vi "NanoStep InitAxis.vi"(6 "CtrlRef":T1 caption="Control Reference", 7 "AxeInv":bool, 8 "error in":errorcluster, 9 "Axis":u16(ring)=1 items=["Axis 0", "Axis 1"], 10 "Input Units":i8(ring) items=["mm", "ps"], 11 "VISA Rsrc":refnum<visa-resource-name>="NANOSTEP") -> (0 "error out":errorcluster, 2 "Pos Out":dbl=0.5)   [LabVIEW 2010]
uses:
  <userlib>/GenProg/WritebyRefBool.vi
  <userlib>/GenProg/ReadbyRefBool.vi
  <userlib>/GenProg/WritebyRefNum.vi
  <userlib>/NanoStep/NanoStep WaitMess.vi
panel:
  out "DatumDone":bool
  out "Canceled":bool
  in  "Annuler":bool
  out "ShowMess":bool
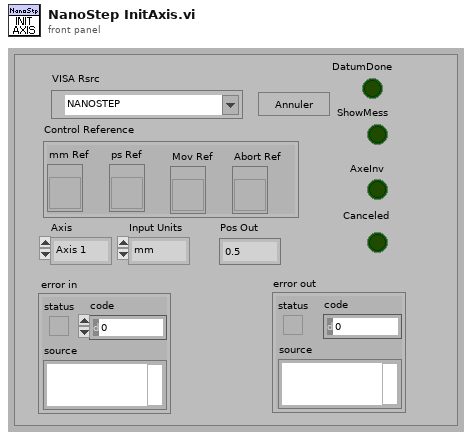
[diagram p1: front panel]
types:
  T1 = cluster{"mm Ref":refnum<vi>, "ps Ref":refnum<vi>, "Mov Ref":refnum<vi>, "Abort Ref":refnum<vi>}
  T2 = enum16{"Clear buffer", "Ack", "Datum", "read position", "end"}
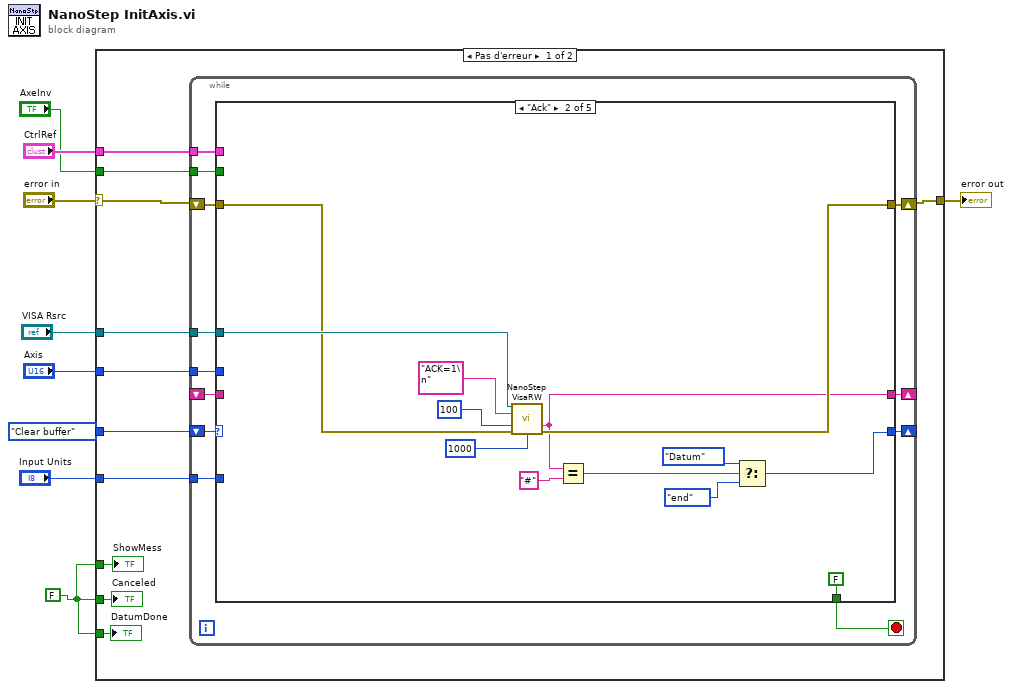
[diagram p0: block diagram]
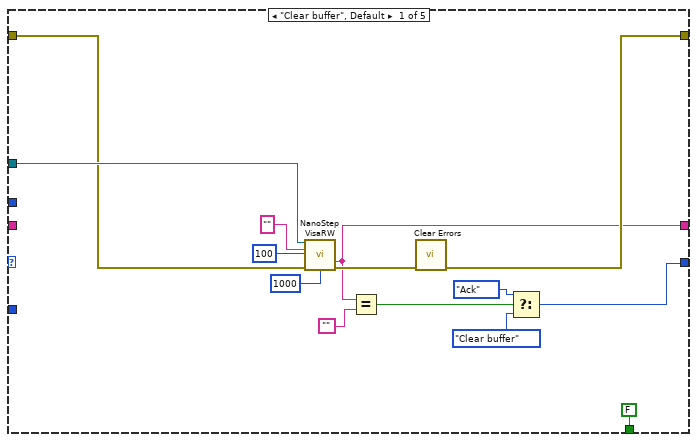
[diagram p2: hidden frame]
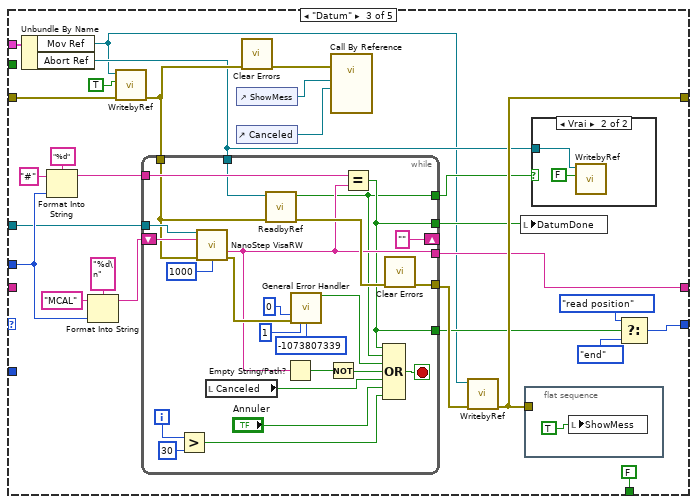
[diagram p3: hidden frame]
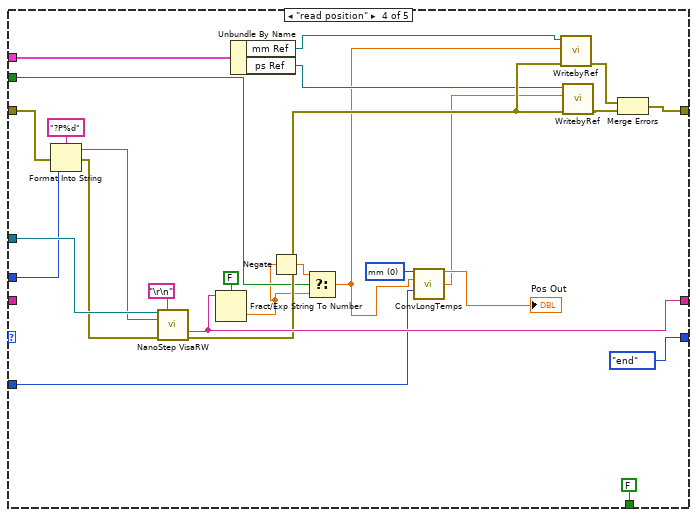
[diagram p5: hidden frame]
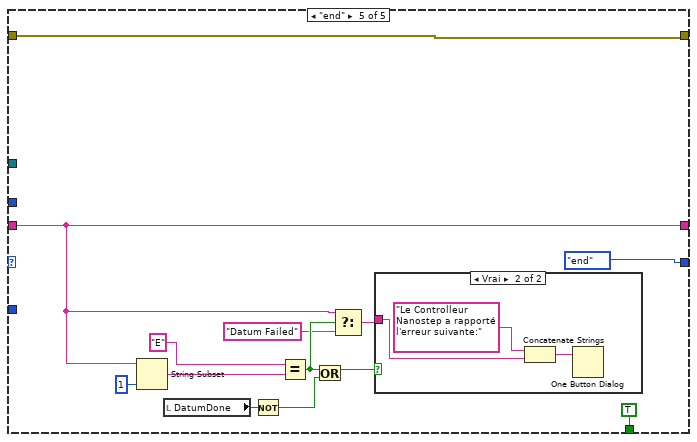
[diagram p6: hidden frame]
diagram:
  w4 = FALSE ("Canceled")
  n1 = case shown="Pas d'erreur" "error in" {
    selector: "error in" -> [w18 w157]
    tunnel: "Axis" -> [w20 _]
    tunnel: [w17 w157] -> w7
    tunnel: T2."Clear buffer" ("Énum") -> [w19 _]
    tunnel: "VISA Rsrc" -> [w16 _]
    tunnel: w4 -> [w15 _]
    tunnel: w4 -> [w14 _]
    tunnel: w4 -> [w13 _]
    tunnel: "CtrlRef" -> [w12 _]
    tunnel: "Input Units" -> [w11 _]
    tunnel: "AxeInv" -> [w10 _]
    frame No Error {
      n2 = while {
        tunnel: w20 -> [w32]
        shift-right: [w28] -> w17
        shift-left: w18 -> [w30]
        tunnel: w16 -> [w29]
        shift-right: [w26] -> _
        shift-left: w19 -> [w31]
        shift-right: [w25] -> _
        shift-left: _ -> [w24]
        tunnel: w12 -> [w23]
        tunnel: w11 -> [w22]
        tunnel: w10 -> [w21]
        stop <- w27 stop-if-true
        n3 = case shown="\"Ack\"" w31 {
          tunnel: w32 -> [_ _ w78 w138 _]
          tunnel: w30 -> [w43 w56 w77 w137 w152]
          tunnel: w29 -> [w46 w59 w72 w140 _]
          tunnel: [w41 w51 w75 w127 w152] -> w28
          tunnel: [FALSE FALSE FALSE FALSE TRUE] -> w27
          tunnel: [w35 w48 w81 T2."end" ("Énum") T2."end" ("Énum")] -> w26
          tunnel: [w34 w47 w71 w131 w145] -> w25
          tunnel: w24 -> [_ _ _ _ w145]
          tunnel: w23 -> [_ _ w64 w125 _]
          tunnel: w22 -> [_ _ _ w121 _]
          tunnel: w21 -> [_ _ _ w118 _]
          frame "Clear buffer", Default {
            n4 = call <userlib>:"NanoStep VisaRW.vi"("VISA Rsrc"=w46, "ChaineCom"="", "Nbcaract"=u32 100, "error in (no error)"=w43, "Timeout(ms)"=u32 1000) -> ("ChaineRep"=w34:string, "error out"=w42:errorcluster)  [unwired: 7 in, 2 out]
            n5 = Equal?(x=w34, y="") -> (x = y?=w38:bool)
            n6 = call <vilib>:"Clear Errors.vi"("error in (no error)"=w42) -> ("error out"=w41:errorcluster)  [unwired: 6 in]
            n7 = Select(t=T2."Ack" ("Énum"), s=w38, f=T2."Clear buffer" ("Énum")) -> (s? t:f=w35:T2)
          }
          frame "Ack" {
            n8 = call <userlib>:"NanoStep VisaRW.vi"("VISA Rsrc"=w59, "ChaineCom"="ACK=1\n", "Nbcaract"=u32 100, "error in (no error)"=w56, "Timeout(ms)"=u32 1000) -> ("ChaineRep"=w47:string, "error out"=w51:errorcluster)  [unwired: 7 in, 2 out]
            n9 = Equal?(x=w47, y="#") -> (x = y?=w54:bool)
            n10 = Select(t=T2."Datum" ("Énum"), s=w54, f=T2."end" ("Énum")) -> (s? t:f=w48:T2)
          }
          frame "Datum" {
            n11 = Unbundle By Name(w64) -> ("Mov Ref"=w60:refnum<vi>, "Abort Ref"=w62:refnum<vi>)
            n12 = Format Into String(format string="%d" ("chaîne de format"), initial string="#" ("y"), w78) -> (resulting string=w74:string)  [unwired: 1 in, 1 out]
            n13 = Format Into String(format string="%d\n" ("chaîne de format"), initial string="MCAL" ("chaîne initiale"), w78) -> (resulting string=w73:string)  [unwired: 1 in, 1 out]
            n14 = call-poly <userlib>:"WritebyRef.vi"("error in"=w77, "Valeur"=TRUE, "Control Ref"=w60) -> ("error out"=w68:errorcluster)  [unwired: 8 in]
            n15 = while {
              tunnel: [w100] -> w70
              tunnel: w72 -> [w112]
              tunnel: [w98] -> w71
              shift-right: [""] -> _
              shift-left: w73 -> [w113]
              tunnel: [w96] -> w66
              tunnel: w74 -> [w97]
              tunnel: [w96] -> w69
              tunnel: w68 -> [w91]
              tunnel: w62 -> [w90]
              tunnel: [w89] -> w63
              i -> [w111]
              stop <- w105 stop-if-true
              n16 = Greater?(x=w111, y=30) -> (0:w92:bool)
              n17 = call <userlib>:"NanoStep VisaRW.vi"("VISA Rsrc"=w112, "ChaineCom"=w113, "error in (no error)"=w91, "Timeout(ms)"=u32 1000) -> ("ChaineRep"=w98:string, "error out"=w107:errorcluster)  [unwired: 8 in, 2 out]
              n18 = local read "Canceled"() -> (w94:bool)
              n19 = call-poly <userlib>:"ReadbyRef.vi"("error in"=w91, "Control Ref"=w90) -> ("error out"=w109:errorcluster, "Valeur"=w89:bool)  [unwired: 8 in]
              n20 = Empty String/Path?(string/path=w98) -> (empty?=w99:bool)
              n21 = call <vilib>:"General Error Handler.vi"("type of dialog (OK msg:1)"=u16 0 ("[exception code]"), "error in (no error)"=w107, "[exception action] (none:0)"=1 ("y"), "[exception code]"=-1073807339) -> ("error?"=w106:bool)  [unwired: 7 in, 4 out]
              n22 = Not(x=w99) -> (.not. x?=w95:bool)
              n23 = Equal?(x=w97, y=w98) -> (x = y?=w96:bool)
              n24 = Compound Arithmetic op=OR(w96, w89, w106, w95, w94, "Annuler", w92) -> (w105:bool)
              n25 = call <vilib>:"Clear Errors.vi"("error in (no error)"=w109) -> ("error out"=w100:errorcluster)  [unwired: 6 in]
            }
            n26 = control-ref of="ShowMess"() -> (w65:refnum<vi>)
            n27 = control-ref of="Canceled"() -> (w67:refnum<vi>)
            n28 = call <vilib>:"Clear Errors.vi"("error in (no error)"=w68) -> ("error out"=w61:errorcluster)  [unwired: 6 in]
            n29 = call-by-ref "?"(error in=w61, "Abort Ref"=w67, "Stop Ref"=w65) -> ()  [unwired: 10 in, 3 out]
            n30 = call-poly <userlib>:"WritebyRef.vi"("error in"=w70, "Control Ref"=w60) -> ("error out"=w75:errorcluster)  [unwired: 9 in]
            n31 = local write "DatumDone"(w66) -> ()
            n32 = flat-sequence {
              tunnel: w75 -> [_]
              frame #0 {
                n33 = local write "ShowMess"(TRUE) -> ()
              }
            }
            n34 = case shown="Vrai" w63 {
              tunnel: w62 -> [_ w88]
              frame False {
              }
              frame True {
                n35 = call-poly <userlib>:"WritebyRef.vi"("Valeur"=FALSE, "Control Ref"=w88) -> ()  [unwired: 9 in, 1 out]
              }
            }
            n36 = Select(t=T2."read position" ("Énum"), s=w69, f=T2."end" ("Énum")) -> (s? t:f=w81:T2)
          }
          frame "read position" {
            w120 = i8 0 items=["mm", "ps"] ("Input Units")
            n37 = Format Into String(format string="?P%d", error in=w137, w138) -> (resulting string=w135:string, error out=w136:errorcluster)  [unwired: 1 in]
            n38 = call <userlib>:"NanoStep VisaRW.vi"("VISA Rsrc"=w140, "EOS (Aucun)"="\r\n", "ChaineCom"=w135, "error in (no error)"=w136) -> ("ChaineRep"=w131:string, "error out"=w128:errorcluster)  [unwired: 8 in, 2 out]
            n39 = Fract/Exp String To Number(use system decimal point (T)=FALSE ("utiliser le séparateur décimal du système (V)"), string=w131) -> (number=w117:dbl)  [unwired: 2 in, 1 out]
            n40 = Unbundle By Name(w125) -> ("mm Ref"=w123:refnum<vi>, "ps Ref"=w124:refnum<vi>)
            n41 = Negate(x=w117) -> (-x=w116:dbl)
            n42 = Select(t=w116, s=w118, f=w117) -> (s? t:f=w115:dbl)
            n43 = call <userlib>:"ConvLongTemps.vi"("Input Units"=w120, "Units Input"=w115, "Output Units"=w121) -> ("Units Output"=→"Pos Out":dbl, "Units ps"=w119:dbl)  [unwired: 9 in, 2 out]
            n44 = call-poly <userlib>:"WritebyRef.vi"("error in"=w128, "Valeur"=w115, "Control Ref"=w123) -> ("error out"=w126:errorcluster)  [unwired: 8 in]
            n45 = call-poly <userlib>:"WritebyRef.vi"("error in"=w128, "Valeur"=w119, "Control Ref"=w124) -> ("error out"=w129:errorcluster)  [unwired: 8 in]
            n46 = Merge Errors(w126, w129) -> (w127:errorcluster)
          }
          frame "end" {
            n47 = String Subset(string=w145, length (rest)=1 ("longueur (reste)")) -> (substring=w149:string)  [unwired: 1 in]
            n48 = local read "DatumDone"() -> (w146:bool)
            n49 = Not(x=w146) -> (.not. x?=w141:bool)
            n50 = Equal?(x="E", y=w149) -> (x = y?=w144:bool)
            n51 = Or(x=w144, y=w141) -> (x .or. y?=w147:bool)
            n52 = Select(t=w145, s=w144, f="Datum Failed") -> (s? t:f=w142:string)
            n53 = case shown="Vrai" w147 {
              tunnel: w142 -> [_ w156]
              frame False {
              }
              frame True {
                n54 = Concatenate Strings("Le Controlleur Nanostep a rapporté l'erreur suivante:", w156) -> (w154:string)
                n55 = One Button Dialog(message=w154) -> ()  [unwired: 1 in, 1 out]
              }
            }
          }
        }
      }
      "Canceled" <- w15
      "ShowMess" <- w14
      "DatumDone" <- w13
    }
    frame Error {
    }
  }
  "error out" <- w7
